vi "crio_SPI_encoder.vi"() -> ()   [LabVIEW 2019]
uses:
  <vilib>/Platform/TimedLoop/XDataNode/timing_clust.ctl
  <vilib>/Platform/TimedLoop/XDataNode/nitl_modes.ctl
  <vilib>/Platform/TimedLoop/XDataNode/wakeup.ctl
  <vilib>/rvi/eio/common/nirviEmuTemplateMethod_errors.vi
  <vilib>/rvi/Emulation/niFpgaSctlEmulationGetInTimedLoop.vi
  <vilib>/rvi/Emulation/niFpgaEmulationReportErrorSimple.vi
  <vilib>/rvi/Emulation/niFpgaGetClockAttributes.vi
  <vilib>/rvi/Emulation/niFpgaCriticalErrorInLSC.vi
  <vilib>/eio/EIOMethodNode/EIOMethodNode.xnode
  <vilib>/Platform/TimedLoop/XDataNode/XDataNode.xnode
  <vilib>/IEDriver/SPIandI2C Slave/FPGA/SPI/Library/SPI Slave FPGA.lvlib
  <vilib>/Platform/TimedLoop/XDataNode/XDNodeRunTimeDep.lvlib
panel:
  in  "stop":bool
  out "Raw Data from Encoder":u32
  in  "data in 2":u32
  in  "data in 1":u32
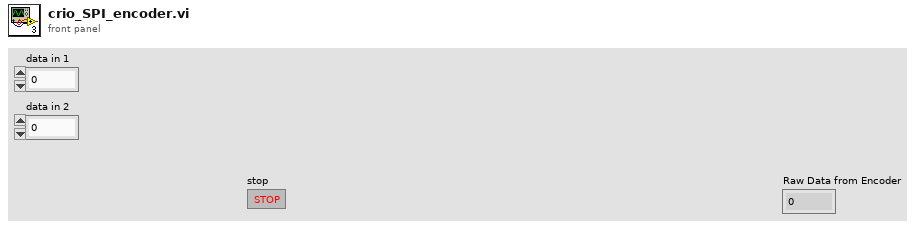
[diagram p1: front panel]
types:
  T1 = typedef "XDNodeRunTimeDep.lvlib/timing_clust.ctl" = cluster{"Expected End [f-1]":u64, "Actual End [f-1]":u64, "Finished Late? [f-1]":bool, "Expected End [i-1]":u64, "Actual End [i-1]":u64, "Finished Late? [i-1]":bool, "Expected Start [i]":u64, "Actual Start [i]":u64, "Expected Start [f]":u64, "Actual Start [f]":u64, "Source Name":string, "Structure Name":string, "Period":i64, "Deadline":i64, "Offset":i64, "Start":i64, "Priority":i32, "Timeout":i32, "Mode":T2, "Wakeup Reason":T3, "Error":errorcluster, "Source Type":string, "Secondary Source Type":string, "Global End Time":u64, "Global Start Time":u64, "Frame Duration":u64, "Iteration Duration":u64, "Assigned CPU":i32, "I/O Scan Engine Mode":u32}
  T2 = typedef "XDNodeRunTimeDep.lvlib/nitl_modes.ctl" = enum32{"No Change", "Process missed periods, maintain original phase", "Discard missed periods, maintain original phase", "Process missed periods, ignore original phase", "Discard missed periods, ignore original phase"}
  T3 = typedef "XDNodeRunTimeDep.lvlib/wakeup.ctl" = enum32{"Normal", "Aborted", "Asynchronous wakeup", "Timing source error", "Timed loop error", "Timeout"}
  T4 = cluster{"SCLK":refnum<k21>, "MISO":refnum<k21>, "MOSI":refnum<k21>, "CS":refnum<k21>}
  T5 = cluster{"API to IP Data":refnum<k21>, "IP to API Data":refnum<k21>, "Configure Register":refnum<k21>}
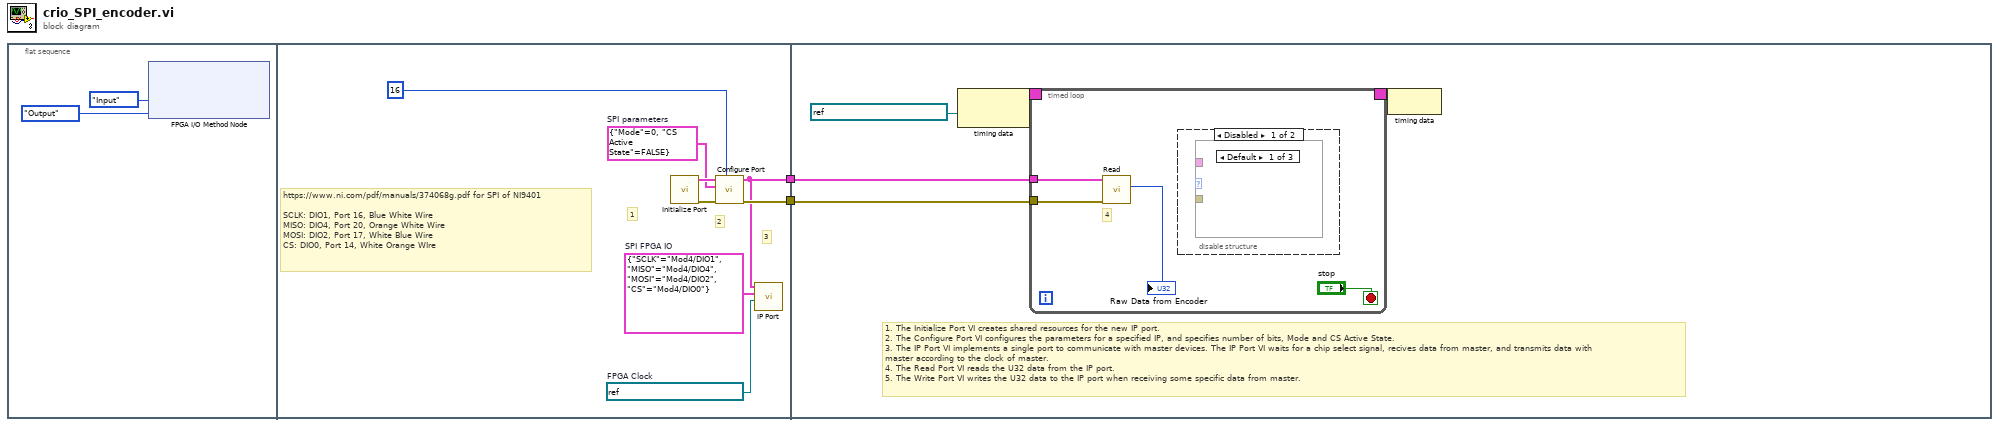
[diagram p0: block diagram]
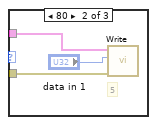
[diagram p2: hidden frame]
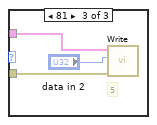
[diagram p3: hidden frame]
diagram:
  n1 = flat-sequence {
    tunnel: [w6] -> w2
    tunnel: [w5] -> w1
    tunnel: w2 -> [w14]
    tunnel: w1 -> [w13]
    frame #0 {
      n2 = xnode "FPGA I/O Method Node"("DIO 7:4"=enum8{"No Change", "Input", "Output"}."Input", "DIO 3:0"=enum8{"No Change", "Input", "Output"}."Output") -> ()  [unwired: 1 in, 1 out]
    }
    frame #1 {
      w9 = cluster{"Mode":i16, "CS Active State":bool} {"Mode"=0, "CS Active State"=FALSE}  # SPI parameters
      w8 = refnum<k21> "40 MHz Onboard Clock"  # FPGA Clock
      w7 = T4 {"SCLK"="Mod4/DIO1", "MISO"="Mod4/DIO4", "MOSI"="Mod4/DIO2", "CS"="Mod4/DIO0"}  # SPI FPGA IO
      # "https://www.ni.com/pdf/manuals/374068g.pdf for SPI of NI9401\n\nSCLK: DIO1, Port 16, Blue White Wire\nMISO: DIO4, Port 20, Orange White Wire\nMOSI: DIO2, Port 17, White Blue Wire\nCS: DIO0, Port 14, White Orange WIre"
      # "3"
      # "2"
      # "1"
      n3 = call <vilib>:"Initialize Port.vi"() -> ("error out"=w11:errorcluster, "private data out"=w12:T5)  [unwired: 9 in]
      n4 = call <vilib>:"Configure Port.vi"("number of bits"=u16 16, "error in (no error)"=w11, "SPI parameters"=w9, "private data in"=w12) -> ("error out"=w6:errorcluster, "private data out"=w5:T5)  [unwired: 5 in, 1 out]
      n5 = call <vilib>:"IP Port.vi"("FPGA clock"=w8, "SPI FPGA IO"=w7, "private data in"=w5) -> ()  [unwired: 9 in]
    }
    frame #2 {
      # "1. The Initialize Port VI creates shared resources for the new IP port.\n2. The Configure Port VI configures the parameters for a specified IP, and specifies number of bits, Mode and CS Active State.\n3. The IP Port VI implements a single port to communicate with master devices. The IP Port VI waits for a chip select signal, recives data from master, and transmits data with \nmaster according to the clock of master.\n4. The Read Port VI reads the U32 data from the IP port. \n5. The Write Port VI writes the U32 data to the IP port when receiving some specific data from master."
      n6 = node-c288(refnum<k21> "40 MHz Onboard Clock" ("Source Name")) -> (w17:T1)
      n7 = timed-loop {
        timing: w17 -> [_]
        timing-out: [_] -> w16
        tunnel: w14 -> [w20]
        tunnel: w13 -> [w19]
        stop <- "stop" stop-if-true
        # "4"
        n8 = call <vilib>:"Read.vi"("error in (no error)"=w20, "private data in"=w19) -> ("data out"=→"Raw Data from Encoder":u32)  [unwired: 5 in, 4 out]
        n9 = disable-structure shown="Disabled" {
          frame Disabled {
            n10 = case shown="Default" {
              selector: _ -> [_ _ _]
              tunnel: _ -> [_ w23 w26]
              tunnel: _ -> [_ w22 w25]
              frame Default {
              }
              frame 80 {
                # "5"
                n11 = call <vilib>:"Write.vi"("error in (no error)"=w22, "data in"="data in 1", "private data in"=w23) -> ()  [unwired: 6 in, 3 out]
              }
              frame 81 {
                # "5"
                n12 = call <vilib>:"Write.vi"("error in (no error)"=w25, "data in"="data in 2", "private data in"=w26) -> ()  [unwired: 6 in, 3 out]
              }
            }
          }
          frame Enabled {
          }
        }
      }
      n13 = node-c288(w16) -> ()
    }
  }
